vi "Write Value at Path.vi"   [LabVIEW 2017, in "Variant Data Manipulation.lvlib"]
uses:
  Variant Data Manipulation.lvlib
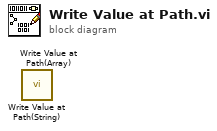
[diagram p0: block diagram]
diagram:
  n1 = call "Write Value at Path(String).vi"() -> ()  [unwired: 10 in, 2 out]
  n2 = call "Write Value at Path(Array).vi"() -> ()  [unwired: 10 in, 2 out]
